vi "ConnectionHeaderReply.vi"(2 "type":string, 3 "Latching":string, 4 "Caller ID":string, 5 "TCPROS Connection Header":string) -> (1 "Connection Response":string)   [LabVIEW 2013]
uses:
  MessageBuilding/Primitives/subs/stringArray.vi
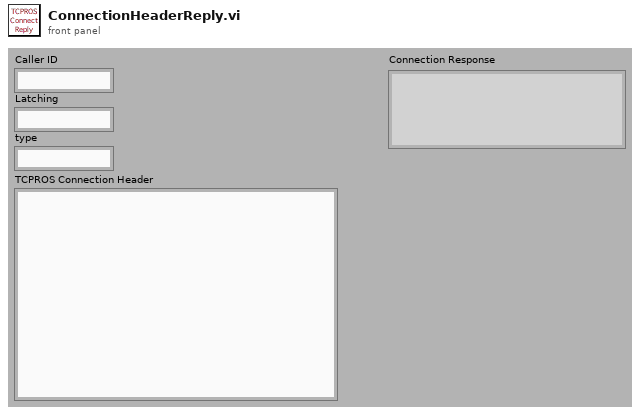
[diagram p1: front panel]
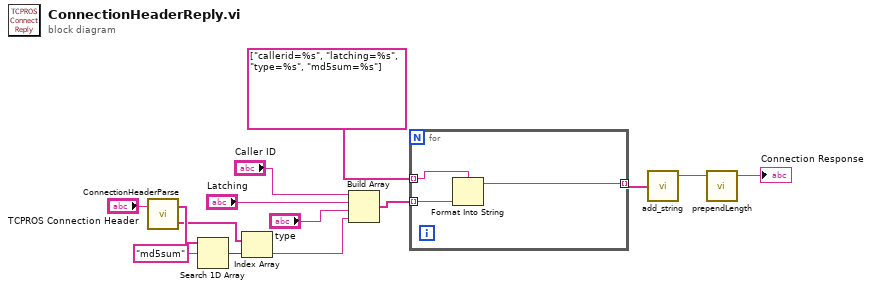
[diagram p0: block diagram]
diagram:
  n1 = call "ConnectionHeaderParse.vi"("TCPROS Connection Header"="TCPROS Connection Header") -> ("Values"=w7:string[], "Fields"=w9:string[])  [unwired: 1 in]
  n2 = Search 1D Array(1D array=w9, element="md5sum") -> (index of element=w6:i32)  [unwired: 1 in]
  n3 = Index Array(array=w7, index=w6) -> (element=w5:string)
  n4 = Build Array("Caller ID", "Latching", "type", w5) -> (w13:string[])
  n5 = for {
    tunnel: string[] ["callerid=%s", "latching=%s", "type=%s", "md5sum=%s"] -> [w17] mode=indexing
    tunnel: w13 -> [w16] mode=indexing
    tunnel: [w15] -> w4 mode=indexing
    n6 = Format Into String(format string=w17, w16) -> (resulting string=w15:string)  [unwired: 2 in, 1 out]
  }
  n7 = call-poly "add_string.vi"("Array"=w4) -> ("msg out"=w2:string)  [unwired: 4 in]
  n8 = call "prependLength.vi"("msg in"=w2) -> ("msg out"=→"Connection Response":string)  [unwired: 4 in]
